vi "Set Limits.vi"(8 "error in (no error)":errorcluster, 9 "Time Limit":dbl, 10 "Round Limit":u32, 11 "Dashboard Panel in":refnum<class "Dashboard Panel.lvclass">) -> (0 "error out":errorcluster, 3 "Dashboard Panel out":refnum<class "Dashboard Panel.lvclass">)   [LabVIEW 2020, in "SB App.lvlib" / "Dashboard Panel.lvclass"]
uses:
  Dashboard Panel.lvclass
  Dashboard Panel.lvclass/Dashboard Panel.ctl
  Limits.ctl
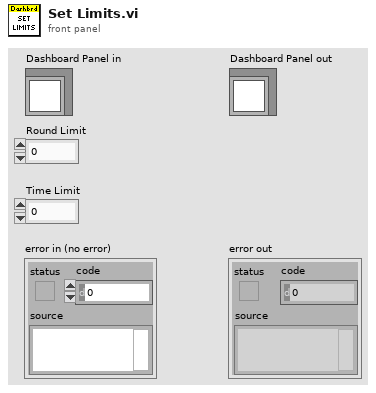
[diagram p1: front panel]
types:
  T1 = typedef "SB App.lvlib/Dashboard Panel.lvclass/Limits.ctl" = cluster{"Round":u32, "Time":dbl}
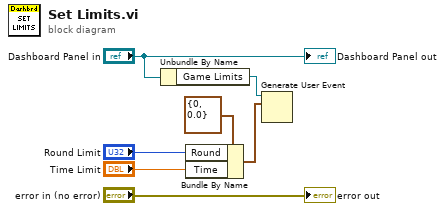
[diagram p0: block diagram]
diagram:
  n1 = Unbundle By Name("Dashboard Panel in") -> ("Game Limits"=w5:refnum<user-event>)
  n2 = Bundle By Name(cluster=T1 {"Round"=0, "Time"=0.0} ("Limits"), "Round"="Round Limit", "Time"="Time Limit") -> (w4:T1)
  n3 = Generate User Event(user event=w5, event data cluster=w4) -> ()  [unwired: 2 in, 2 out]
  "error out" <- "error in (no error)"
  "Dashboard Panel out" <- "Dashboard Panel in"
